vi "RegForSpecificMsg.vi"(6 "_Msg-Filter":refnum<class "_Msg-Filter.lvclass">, 8 "error in (no error)":errorcluster, 9 "MailboxManager":refnum<class "Message Enqueuer.lvclass">, 10 "MailBoxMessage":refnum<class "MailBoxMessage.lvclass">, 11 "MailboxClient in":refnum<class "MailboxClient.lvclass">) -> (0 "error out":errorcluster, 3 "MailboxClient out":refnum<class "MailboxClient.lvclass">)   [LabVIEW 2020, in "MailboxClient.lvlib" / "MailboxClient.lvclass"]
uses:
  MailboxClient.lvclass
  MailboxManager/MailboxManager Messages/RegisterForMessageSpecificType Msg/RegisterForMessageSpecificType Msg.lvclass
  <vilib>/ActorFramework/Actor/Actor.lvclass
  C:/Program Files (x86)/National Instruments/LabVIEW 2020/vi.lib/ActorFramework/Actor/Actor.lvclass
  C:/Users/taylo/Projects/LabVIEW/ActorMailbox/MailboxClient/MailboxClient/MailboxClient.lvclass
  MailboxManager/_Msg-Filter/_Msg-Filter.lvclass
  MailboxManager/MailBoxMessage/MailBoxMessage.lvclass
  <vilib>/ActorFramework/Message Enqueuer/Message Enqueuer.lvclass
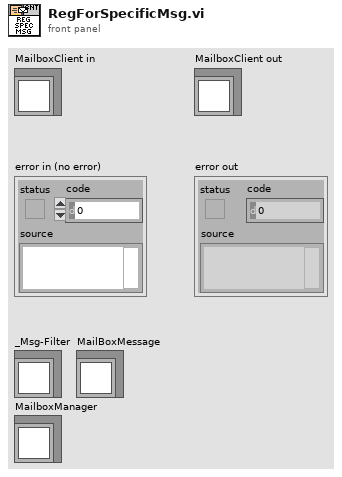
[diagram p1: front panel]
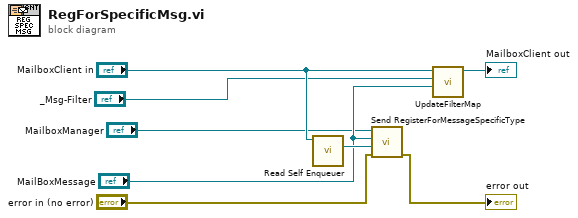
[diagram p0: block diagram]
diagram:
  n1 = call <vilib>:"Read Self Enqueuer.vi"("Actor"="MailboxClient in") -> ("Self Enqueuer"=w8:refnum<class "Message Enqueuer.lvclass">)  [unwired: 10 in]
  n2 = call "Send RegisterForMessageSpecificType.vi"("error in (no error)"="error in (no error)", "Message Enqueuer 2"=w8, "MailBoxMessage"="MailBoxMessage", "Message Enqueuer"="MailboxManager") -> ("error out"=→"error out":errorcluster)  [unwired: 6 in, 1 out]
  n3 = call "UpdateFilterMap.vi"("MailBoxMessage"="MailBoxMessage", "_Msg-Filter"="_Msg-Filter", "MailboxClient in"="MailboxClient in") -> ("MailboxClient out"=→"MailboxClient out":refnum<class "MailboxClient.lvclass">)  [unwired: 8 in]
